vi "imp_test_v12_p.vi"() -> ()   [LabVIEW 2014]
uses:
  <vilib>/LabVIEW Targets/FPGA/cRIO/shared/nicrio_ModuleControls/nicrio_cRIO-9237_DataRatesRing.ctl
  <vilib>/LabVIEW Targets/FPGA/cRIO/shared/nicrio_ModuleControls/nicrio_cRIO-9237_ExcitationVoltageRing.ctl
  <vilib>/rvi/FXPMathLib/FxpSinAndCos/subVIs/nifxpmath_SinAndCos_SimConfig.ctl
  <vilib>/rvi/FXPMathLib/FxpSqrt/subVIs/nifxpmath_Sqrt_SimConfig.ctl
  <vilib>/fxp/LVFixedPointOverflowPolicyTypeDef.ctl
  <vilib>/rvi/FXPMathLib/FxpAtan2/subVIs/nifxpmath_Atan2_SimConfig.ctl
  <vilib>/rvi/Emulation/niFpgaGetClockAttributes.vi
  <vilib>/rvi/Emulation/niFpgaSctlEmulationGetInTimedLoop.vi
  <vilib>/rvi/Emulation/niFpgaEmulationReportErrorSimple.vi
  <vilib>/rvi/Emulation/niFpgaProcessEmulError.vi
  <vilib>/rvi/interface/RandomDataEmulation/nirviRandomDataMultiElementFPGAFIFO.vi
  <instcachedir>/0/nirviRandomDataMultiElementFPGAFIFO_AD0CFC12EF974623A9C2E4184BC062B2.lvgen/nirviRandomDataMultiElementFPGAFIFO_AD0CFC12EF974623A9C2E4184BC062B2_028.vi
  <vilib>/rvi/interface/RandomDataEmulation/niFpgaRandomDataHandleErrors.vi
  <vilib>/rvi/Emulation/niFpgaCriticalErrorInLSC.vi
  <vilib>/rvi/FXPMathLib/FxpSinAndCos/simVIs/DllFxpSinAndCosTemp_sub.vi
  <vilib>/rvi/eio/common/nirviEmuTemplateMethod_errors.vi
  <vilib>/rvi/FXPMathLib/FxpSqrt/simVIs/DllSqrtTemp_sub.vi
  <vilib>/rvi/FXPMathLib/FxpAtan2/simVIs/DllFxpAtan2Temp_sub.vi
  <vilib>/rvi/eio/common/nirviEmuTemplatePropertySet_errors.vi
  <vilib>/rvi/DataTransferAndStorage/Container/XNode/niFpgaContainer.xnode
  <vilib>/rvi/interface/RandomDataEmulation/nirviRandomDataFpgaMultiElementTemplate.vi
  <vilib>/rvi/Analysis/measure/butterworth/XNode/niFpgaButterworthFilter.xnode
  <vilib>/rvi/FXPMathLib/FxpSinAndCos/XNode/nifxpmath_SinAndCos.xnode
  <vilib>/eio/EIONode/EIONode.xnode
  <vilib>/rvi/FXPMathLib/FxpSqrt/XNode/nifxpmath_Sqrt.xnode
  <vilib>/rvi/FXPMathLib/FxpAtan2/XNode/nifxpmath_Atan2.xnode
  <vilib>/eio/EIOPropertyNode/EIOPropertyNode.xnode
  <vilib>/rvi/eio/common/nirviEmuTemplatePropertyGet_errors.vi
  <vilib>/rvi/eio/common/nirviEmuTemplatePropertyGet_noerrors.vi
  <vilib>/rvi/eio/common/nirviEmuTemplatePropertySet_noerrors.vi
panel:
  out "(b^2-ac)p3":fxp<+/-,64,35>
  out "(b^2-ac)p2":fxp<+/-,64,34>
  in  "kv_p (Nm/rad)":fxp<+/-,32,7>
  out "tau_p (Nm)":fxp<+/-,53,16>
  out "theta3p (rad)":fxp<+/-,19,5>
  out "theta2p (rad)":fxp<+/-,16,2>
  out "r4p":fxp<+/-,32,9>
  in  "force_lim":fxp<+,22,9>
  in  "Mavg f loop(uSec)":u32
  in  "F_Threshold_p":fxp<+,12,4>
  out "omega_p (Mavg)":fxp<+/-,36,13>
  out "Dp_d (Mavg)":fxp<+/-,36,13>
  out "omega_p2 (Mavg)":fxp<+/-,36,14>
  out "Dp2_d (Mavg)":fxp<+/-,36,14>
  in  "mt0_p2":u32
  out "Dp_d (Mavg w. f.)":fxp<+/-,36,14>
  in  "Dp_d (Mavg) coeff.":i32[](array[numeric])=[946630756, 63555534]
  out "omega_p (Mavg w. f)":fxp<+/-,36,14>
  in  "omega_P(Mavg) coeff.":i32[](array[numeric])=[946630756, 63555534]
  out "PID (kHz)":fxp<+/-,20,10>
  in  "Set 6":bool
  in  "Set 5":bool
  in  "Set 4":bool
  in  "Set 3":bool
  in  "Set 2":bool
  in  "Set 1":bool
  out "Dp1_d (T)":fxp<+/-,36,13>
  out "omega_p1 (T)":fxp<+/-,36,13>
  out "Dp2_d (T)":fxp<+/-,36,13>
  out "omega_p2 (T)":fxp<+/-,36,13>
  out "mt_omega_p2":u32
  out "Encoder Position_p2":i32
  out "D_p2":fxp<+/-,32,7>
  out "rad_p2":fxp<+/-,33,20>
  out "D_p1":fxp<+/-,32,7>
  out "rad_p1":fxp<+/-,33,20>
  out "Encoder Position_p1":i32
  out "Dp1_d (Mavg)":fxp<+/-,36,14>
  out "omega_p1 (Mavg)":fxp<+/-,36,14>
  in  "Dp_d_M_avg_Tc (uSec)":i32
  out "Dp_d (T)":fxp<+/-,36,13>
  out "omega_p (T)":fxp<+/-,36,13>
  in  "Vp. Est.":i16(ring) items=["T", "Mavg", "Mavg w. f."]
  in  "Mag. factor_p":fxp<+/-,20,3>
  in  "Mag. encoder_p":bool
  in  "Belt_out_p":fxp<+/-,7,7>
  in  "Belt_in_p":fxp<+/-,6,6>
  out "Fp_dc":fxp<+/-,32,10>
  in  "Zero_p":bool
  in  "mt0_p1":u32
  in  "Encoder reset":bool
  out "fpt_d":fxp<+/-,36,18>
  out "Dp_error_dd":fxp<+/-,36,16>
  out "Dp_error_d":fxp<+/-,33,8>
  in  "Dp_dd coeff.":i32[](array[numeric])=[946630756, 63555534]
  out "Dp_dd":fxp<+/-,36,25>
  out "dFp_PID":fxp<+/-,36,18>
  in  "dFp_PID coeff.":i32[](array[numeric])=[946630756, 63555534]
  out "fpt_i":fxp<+/-,34,18>
  in  "Bv_p":fxp<+/-,22,8>
  in  "Kv_p":fxp<+/-,26,7>
  out "Dp_error":fxp<+/-,22,7>
  out "Dpr_sin":fxp<+/-,22,7>
  in  "Sin offset_p":fxp<+/-,22,7>
  in  "Sin magnitude_p":fxp<+/-,21,6>
  out "Dpr_sin_dd":fxp<+/-,35,20>
  out "Dpr_sin_d":fxp<+/-,33,15>
  out "Sin omega_p":fxp<+/-,34,9>
  in  "Sin wave freq._p (Hz)":fxp<+/-,32,6>
  in  "Dpr_step":fxp<+/-,22,7>
  out "Dpr_for":fxp<+/-,22,7>
  in  "Command_p":i16(ring) items=["Step", "Sine"]
  in  "Ki_p":fxp<+/-,30,9>
  out "Fp_PID":fxp<+/-,36,16>
  in  "fp_tolorance":fxp<+,22,6>
  out "fp_tilde":fxp<+/-,33,10>
  in  "Kd_p":fxp<+/-,30,9>
  in  "Kp_p":fxp<+/-,32,13>
  out "Fr_p":fxp<+/-,32,10>
  in  "S/F coeff_p":fxp<+/-,25,-10>
  out "va_p":fxp<+/-,36,7>
  out "vb_p":fxp<+/-,37,8>
  out "vq_p_F":fxp<+/-,20,5> format="%.57g"
  out "vd_p_F":fxp<+/-,20,5>
  in  "dFp_add":bool
  in  "Stop motor_p":bool
  out "Force_p":fxp<+/-,32,10>
  in  "Strain selection_p":i16(ring) items=["Raw", "Avg.8", "Avg.8 w. filter"]
  out "Strain_p (Avg8 w. f)":fxp<+/-,36,8>
  in  "Strain_p Avg.8 coeff.":i32[](array[numeric])=[946630756, 63555534]
  out "Strain_p (Avg8)":fxp<+/-,36,4>
  out "Raw Strain_p":fxp<+/-,36,4>
  out "Mod6/AI3":fxp<+/-,36,4>
  in  "Strain gage reset_p":bool
  out "Dp_d (mm/s)":fxp<+/-,36,13>
  out "omega_p (rad/s)":fxp<+/-,36,13>
  out "mt_omega_p1":u32
  out "rad_p(NrTheta)":fxp<+/-,33,20>
  out "D_p(mm)":fxp<+/-,32,7>
  out "Encoder Position_p":i32
  in  "Encoder reset_p":bool
  out "Time now(s)":fxp<+,52,14>
  in  "Drive mode":i16(ring) items=["Backward", "Forward", "Imp", "Imp(tau2theta)"]
  in  "Ini coe.":bool
  out "Loop rate (kHz)":fxp<+/-,36,7>
  in  "Stop (Strain)":bool
  in  "Excitation Voltage":T1 items=["2.5 Volts", "3.3 Volts", "5.0 Volts", "10.0 Volts", "External Excitation"]
  in  "Data Rate":T2=1 items=["50.000 kS/s (NI 9237)"=1, "25.000 kS/s (NI 9237)"=2, "16.667 kS/s (NI 9237)"=3, "12.500 kS/s (NI 9237)"=4, "10.000 kS/s (NI 9237)"=5, "8.333 kS/s (NI 9237)"=6, "7.143 kS/s (NI 9237)"=7, "6.250 kS/s (NI 9237)"=8, "5.556 kS/s (NI 9237)"=9, "5.000 kS/s (NI 9237)"=10, "4.545 kS/s (NI 9237)"=11, "4.167 kS/s (NI 9237)"=12, "3.846 kS/s (NI 9237)"=13, "3.571 kS/s (NI 9237)"=14, "3.333 kS/s (NI 9237)"=15, "3.125 kS/s (NI 9237)"=16, "2.941 kS/s (NI 9237)"=17, "2.778 kS/s (NI 9237)"=18, "2.632 kS/s (NI 9237)"=19, "2.500 kS/s (NI 9237)"=20, "2.381 kS/s (NI 9237)"=21, "2.273 kS/s (NI 9237)"=22, "2.174 kS/s (NI 9237)"=23, "2.083 kS/s (NI 9237)"=24, "2.000 kS/s (NI 9237)"=25, "1.923 kS/s (NI 9237)"=26, "1.852 kS/s (NI 9237)"=27, "1.786 kS/s (NI 9237)"=28, "1.724 kS/s (NI 9237)"=29, "1.667 kS/s (NI 9237)"=30, "1.613 kS/s (NI 9237)"=31]
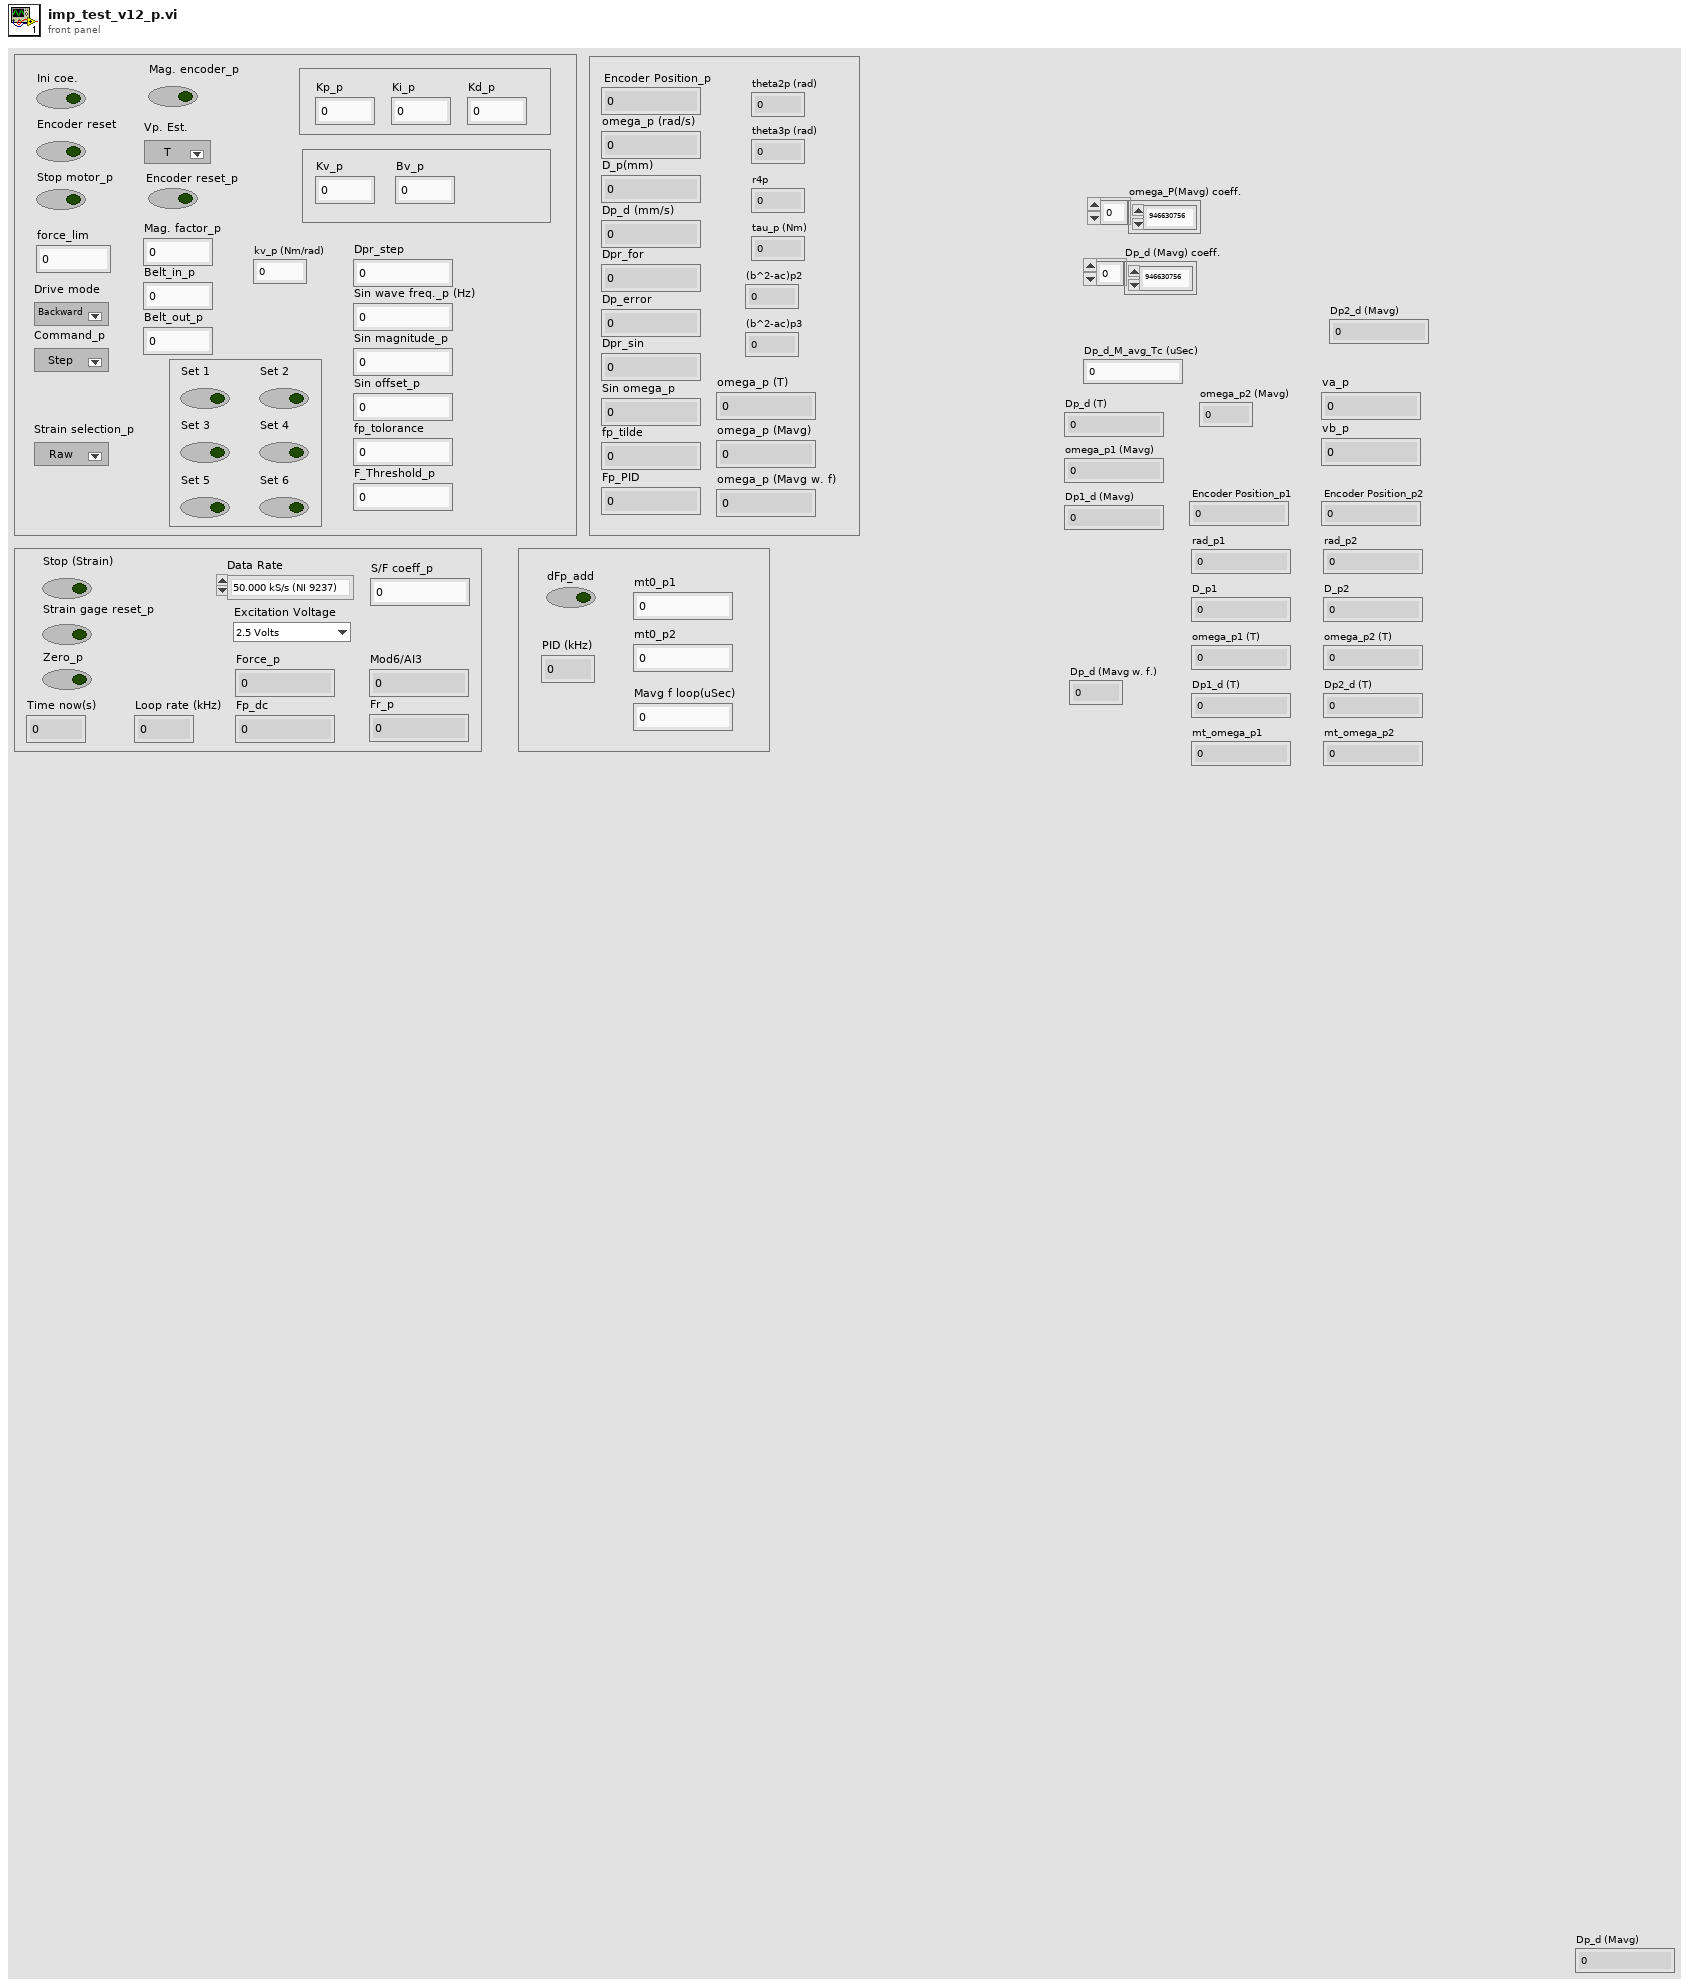
[diagram p1: front panel]
types:
  T1 = typedef "nicrio_cRIO-9237_ExcitationVoltageRing.ctl" = u8
  T2 = typedef "nicrio_cRIO-9237_DataRatesRing.ctl" = u8
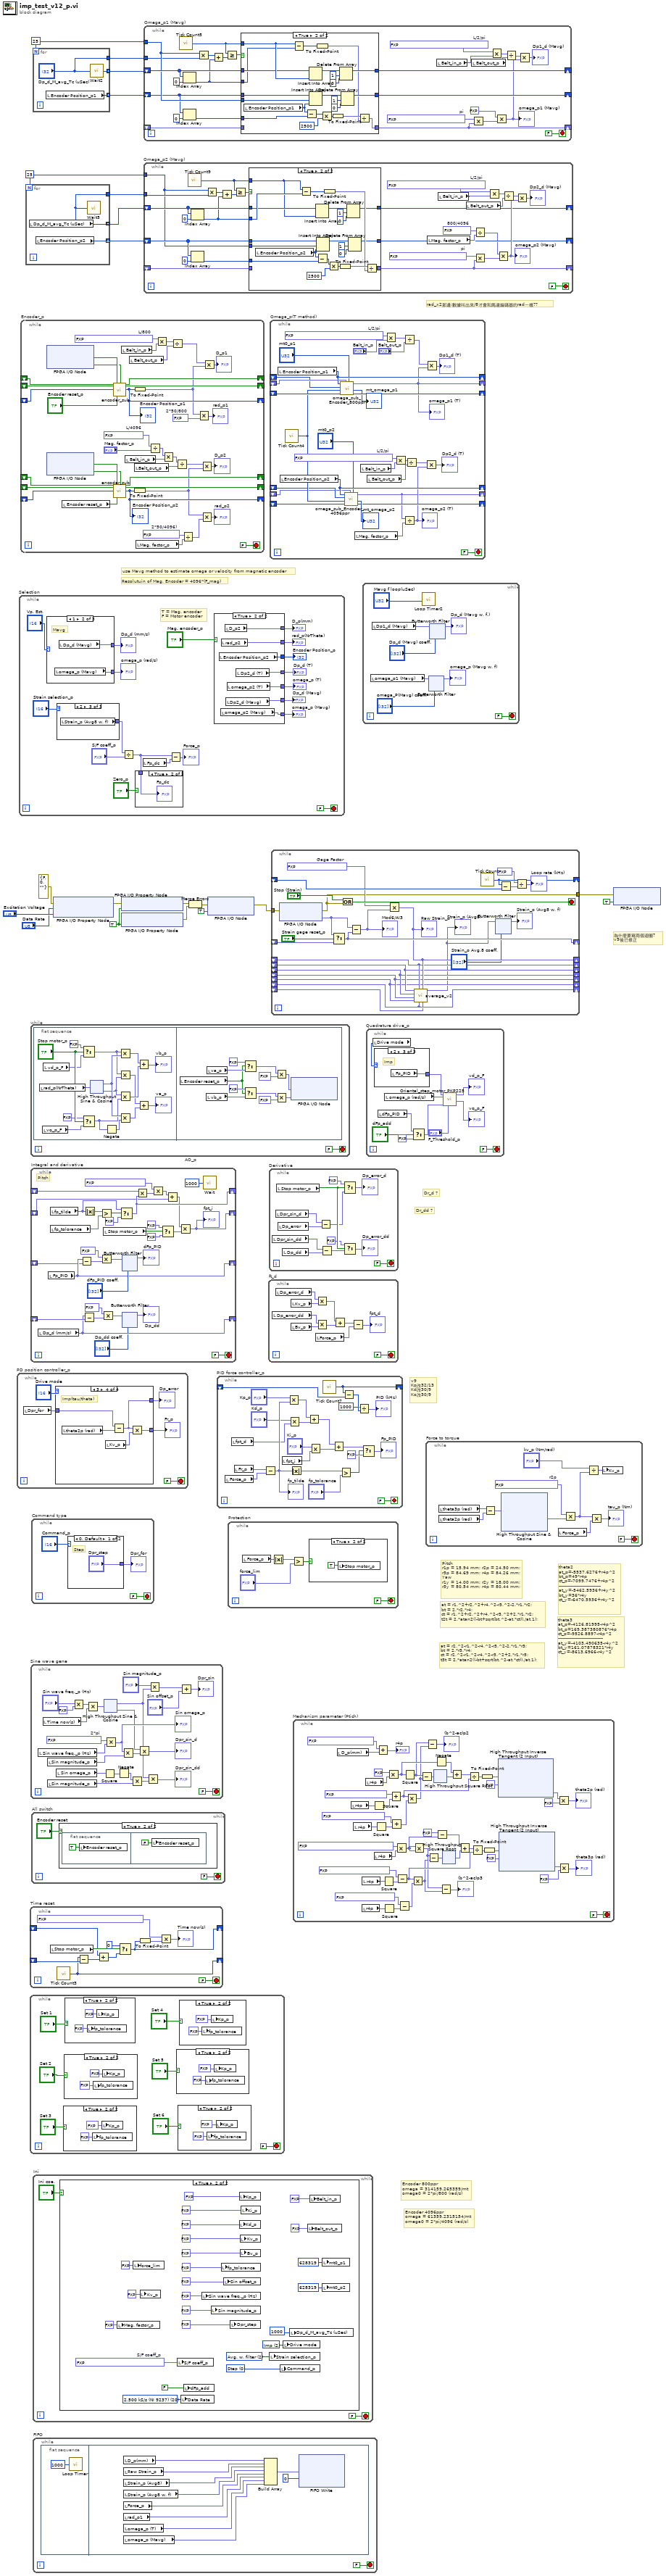
[diagram p0: block diagram]
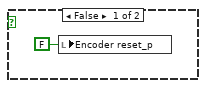
[diagram p11: hidden frame]
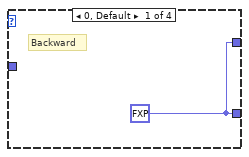
[diagram p12: hidden frame]
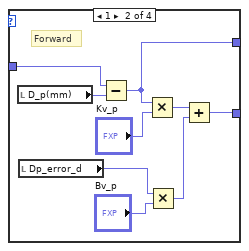
[diagram p13: hidden frame]
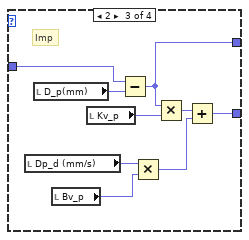
[diagram p14: hidden frame]
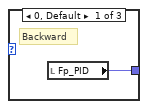
[diagram p15: hidden frame]
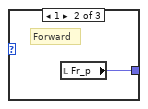
[diagram p16: hidden frame]
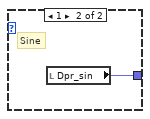
[diagram p17: hidden frame]
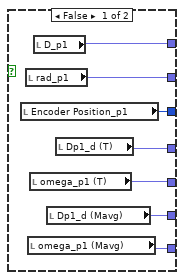
[diagram p18: hidden frame]
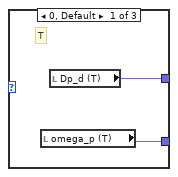
[diagram p19: hidden frame]
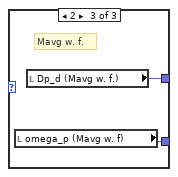
[diagram p20: hidden frame]
diagram:
  w2 = 25
  w8 = 25
  w13 = TRUE ("Half-Bridge Enable")
  # "theta3\nat_p=-4126.81995-r4p^2\nbt_p=169.387380876*r4p\nct_p=-9526.8897-r4p^2\n-------------------------------\nat_y=-4103.490635-r4y^2\nbt_y=161.07878321*r4y\nct_y=-8613.6966-r4y^2"
  # "at = r2.^2-r1.^2-r4.^2-r3.^2-2.*r1.*r3;\nbt = 2.*r3.*r4;\nct = r2.^2-r1.^2-r4.^2-r3.^2+2.*r1.*r3;\nt3t = 2.*atan2((-bt+sqrt(bt.^2-at.*ct))./at,1);"
  # "theta2\nat_p=-5537.6276+r4p^2\nbt_p=49*r4p\nct_p=-7099.7476+r4p^2\n-----------------------------\nat_y=-5462.5936+r4y^2\nbt_y=36*r4y\nct_y=-6470.5936+r4y^2"
  # "Pitch\nr1p = 15.94 mm; r2p = 24.50 mm;\nr3p = 84.69 mm; r4p = 84.26 mm;\nYaw\nr1y = 14.00 mm; r2y = 18.00 mm;\nr3y = 80.54 mm; r4p = 80.44 mm;"
  # "at = r1.^2+r2.^2+r4.^2-r3.^2-2.*r1.*r2;\nbt = 2.*r2.*r4;\nct = r1.^2+r2.^2+r4.^2-r3.^2+2.*r1.*r2;\nt2t = 2.*atan2((-bt+sqrt(bt.^2-at.*ct))./at,1);"
  # "rad_x2那邊:數據叫出來/8才會和馬達編碼器的rad一樣??"
  # "Encoder 4096ppr\nomega = 61359.2315154/mt\nomega0 = 2*pi/4096 (rad/s)"
  # "Encoder 800ppr\nomega = 314159.265359/mt\nomega0 = 2*pi/800 (rad/s)"
  # "v9\nKp改32/13\nKd改30/9\nKo改30/9"
  # "Resolutuin of Mag. Encoder = 4096*(F_mag)"
  # "use Mavg method to estimate omega or velocity from magnetic encoder"
  # "為什麼要寫兩個迴圈?\nv9後已修正"
  # "Dr_dd ?"
  # "Dr_d ?"
  n1 = while "PD position controller_p" {
    stop <- FALSE stop-if-true
    n2 = local read "Dpr_for"() -> (w21:fxp<+/-,22,7>)
    n3 = case shown="3" "Drive mode" {
      tunnel: [w26 w30 w37 w45] -> w25
      tunnel: [w26 w28 w42 w47] -> w22
      tunnel: w21 -> [_ w27 w36 w46]
      frame 0, Default {
        w26 = fxp<+/-,62,19> 0.0
        # "Backward"
      }
      frame 1 {
        # "Forward"
        n4 = local read "D_p(mm)"() -> (w35:fxp<+/-,32,7>)
        n5 = local read "Dp_error_d"() -> (w29:fxp<+/-,33,8>)
        n6 = Subtract(x=w27, y=w35) -> (x-y=w28:fxp<+/-,33,8>)
        n7 = Multiply(x=w28, y="Kv_p") -> (x*y=w32:fxp<+/-,58,14>)
        n8 = Multiply(x=w29, y="Bv_p") -> (x*y=w31:fxp<+/-,55,16>)
        n9 = Add(x=w32, y=w31) -> (x+y=w30:fxp<+/-,60,16>)
      }
      frame 2 {
        # "Imp"
        n10 = local read "Dp_d (mm/s)"() -> (w40:fxp<+/-,36,13>)
        n11 = local read "D_p(mm)"() -> (w43:fxp<+/-,32,7>)
        n12 = local read "Bv_p"() -> (w39:fxp<+/-,22,8>)
        n13 = local read "Kv_p"() -> (w44:fxp<+/-,26,7>)
        n14 = Subtract(x=w36, y=w43) -> (x-y=w42:fxp<+/-,33,8>)
        n15 = Multiply(x=w40, y=w39) -> (x*y=w38:fxp<+/-,58,21>)
        n16 = Multiply(x=w42, y=w44) -> (x*y=w41:fxp<+/-,58,14>)
        n17 = Add(x=w41, y=w38) -> (x+y=w37:fxp<+/-,64,21>)
      }
      frame 3 {
        # "Imp(tau/theta)"
        n18 = local read "theta2p (rad)"() -> (w48:fxp<+/-,16,2>)
        n19 = local read "Kv_p"() -> (w49:fxp<+/-,26,7>)
        n20 = Subtract(x=w46, y=w48) -> (x-y=w47:fxp<+/-,23,8>)
        n21 = Multiply(x=w47, y=w49) -> (x*y=w45:fxp<+/-,48,14>)
      }
    }
    "Fr_p" <- w25
    "Dp_error" <- w22
  }
  n22 = while "Selection" {
    stop <- FALSE stop-if-true
    # "T = Mag. encoder\nF = Motor encoder"
    n23 = case shown="1" "Vp. Est." {
      tunnel: [w84 w85 w88] -> w60
      tunnel: [w83 w86 w87] -> w61
      frame 0, Default {
        # "T"
        n24 = local read "omega_p (T)"() -> (w84:fxp<+/-,36,13>)
        n25 = local read "Dp_d (T)"() -> (w83:fxp<+/-,36,13>)
      }
      frame 1 {
        # "Mavg"
        n26 = local read "omega_p (Mavg)"() -> (w85:fxp<+/-,36,13>)
        n27 = local read "Dp_d (Mavg)"() -> (w86:fxp<+/-,36,13>)
      }
      frame 2 {
        # "Mavg w. f."
        n28 = local read "omega_p (Mavg w. f)"() -> (w88:fxp<+/-,36,14>)
        n29 = local read "Dp_d (Mavg w. f.)"() -> (w87:fxp<+/-,36,14>)
      }
    }
    "Dp_d (mm/s)" <- w61
    "omega_p (rad/s)" <- w60
    n30 = case shown="2" "Strain selection_p" {
      tunnel: [w90 w91 w92] -> w67
      frame 0, Default {
        n31 = local read "Raw Strain_p"() -> (w90:fxp<+/-,36,4>)
      }
      frame 1 {
        n32 = local read "Strain_p (Avg8)"() -> (w91:fxp<+/-,36,4>)
      }
      frame 2 {
        n33 = local read "Strain_p (Avg8 w. f)"() -> (w92:fxp<+/-,36,8>)
      }
    }
    n34 = Divide(x=w67, y="S/F coeff_p") -> (x/y=w64:fxp<+/-,32,10>)
    n35 = case shown="True" "Zero_p" {
      tunnel: w64 -> [_ w89]
      frame False {
      }
      frame True {
        "Fp_dc" <- w89
      }
    }
    n36 = local read "Fp_dc"() -> (w62:fxp<+/-,32,10>)
    n37 = Subtract(x=w64, y=w62) -> (x-y=→"Force_p":fxp<+/-,33,11>)
    n38 = case shown="True" "Mag. encoder_p" {
      tunnel: [w75 w82] -> w56
      tunnel: [w74 w81] -> w57
      tunnel: [w73 w80] -> w58
      tunnel: [w71 w79] -> w54
      tunnel: [w72 w78] -> w53
      tunnel: [w70 w76] -> w52
      tunnel: [w69 w77] -> w51
      frame False {
        n39 = local read "Encoder Position_p1"() -> (w73:i32)
        n40 = local read "rad_p1"() -> (w74:fxp<+/-,33,20>)
        n41 = local read "omega_p1 (Mavg)"() -> (w69:fxp<+/-,36,14>)
        n42 = local read "omega_p1 (T)"() -> (w71:fxp<+/-,36,13>)
        n43 = local read "D_p1"() -> (w75:fxp<+/-,32,7>)
        n44 = local read "Dp1_d (Mavg)"() -> (w70:fxp<+/-,36,14>)
        n45 = local read "Dp1_d (T)"() -> (w72:fxp<+/-,36,13>)
      }
      frame True {
        n46 = local read "Encoder Position_p2"() -> (w80:i32)
        n47 = local read "omega_p2 (Mavg)"() -> (w77:fxp<+/-,36,14>)
        n48 = local read "rad_p2"() -> (w81:fxp<+/-,33,20>)
        n49 = local read "D_p2"() -> (w82:fxp<+/-,32,7>)
        n50 = local read "Dp2_d (Mavg)"() -> (w76:fxp<+/-,36,14>)
        n51 = local read "omega_p2 (T)"() -> (w79:fxp<+/-,36,13>)
        n52 = local read "Dp2_d (T)"() -> (w78:fxp<+/-,36,13>)
      }
    }
    "D_p(mm)" <- w56
    "rad_p(NrTheta)" <- w57
    "Encoder Position_p" <- w58
    "Dp_d (T)" <- w53
    "omega_p (T)" <- w54
    "Dp_d (Mavg)" <- w52
    "omega_p (Mavg)" <- w51
  }
  n53 = while "Encoder_p" {
    shift-right: [w130] -> _
    shift-left: _ -> [w129]
    shift-right: [w131] -> _
    shift-left: _ -> [w128]
    shift-right: [w125] -> _
    shift-left: _ -> [w127]
    shift-right: [w116] -> _
    shift-left: _ -> [w115]
    shift-right: [w117] -> _
    shift-left: _ -> [w118]
    shift-right: [w112] -> _
    shift-left: _ -> [w113]
    stop <- FALSE stop-if-true
    w108 = fxp<+/-,20,-5> 0.00048828125  # L/4096
    w106 = fxp<+/-,16,1> 0.0244140625  # 2*50/4096)
    w124 = fxp<+/-,20,-5> 0.002499997615814209  # L/800
    w98 = fxp<+/-,16,1> 0.125  # 2*50/800
    n54 = xnode "FPGA I/O Node"() -> ("Mod7/DIO0"=w133:bool, "Mod7/DIO1"=w132:bool)  [unwired: 2 in, 2 out]
    n55 = xnode "FPGA I/O Node"() -> ("Mod7/DIO4"=w120:bool, "Mod7/DIO5"=w119:bool)  [unwired: 2 in, 2 out]
    n56 = local read "Encoder reset_p"() -> (w114:bool)
    n57 = call "encoder_sub.vi"("A_pre"=w129, "B_pre"=w128, "Encoder Position_pre"=w127, "A input"=w133, "Encoder Position Reset"="Encoder reset_p", "B input"=w132) -> ("A"=w130:bool, "B"=w131:bool, "Encoder Position (Counts)"=w125:i32)  [unwired: 19 in]
    "Encoder Position_p1" <- w125
    n58 = call "encoder_sub.vi"("A_pre"=w115, "B_pre"=w118, "Encoder Position_pre"=w113, "A input"=w120, "Encoder Position Reset"=w114, "B input"=w119) -> ("A"=w116:bool, "B"=w117:bool, "Encoder Position (Counts)"=w112:i32)  [unwired: 19 in]
    "Encoder Position_p2" <- w112
    n59 = local read "Belt_in_p"() -> (w123:fxp<+/-,6,6>)
    n60 = local read "Belt_in_p"() -> (w109:fxp<+/-,6,6>)
    n61 = local read "Belt_out_p"() -> (w121:fxp<+/-,7,7>)
    n62 = To Fixed-Point(number=w112) -> (fixed-point=w94:fxp<+/-,32,32>)  [unwired: 1 in]
    n63 = To Fixed-Point(number=w125) -> (fixed-point=w99:fxp<+/-,32,32>)  [unwired: 1 in]
    n64 = local read "Belt_out_p"() -> (w111:fxp<+/-,7,7>)
    n65 = local read "Mag. factor_p"() -> (w105:fxp<+/-,20,3>)
    n66 = Divide(x=w108, y="Mag. factor_p") -> (x/y=w107:fxp<+/-,41,13>)
    n67 = Multiply(x=w124, y=w123) -> (x*y=w122:fxp<+/-,26,1>)
    n68 = Multiply(x=w107, y=w109) -> (x*y=w110:fxp<+/-,46,18>)
    n69 = Divide(x=w122, y=w121) -> (x/y=w101:fxp<+/-,33,1>)
    n70 = Divide(x=w110, y=w111) -> (x/y=w96:fxp<+/-,53,18>)
    n71 = Divide(x=w106, y=w105) -> (x/y=w93:fxp<+/-,37,5>)
    n72 = Multiply(x=w99, y=w98) -> (x*y=→"rad_p1":fxp<+/-,33,20>)
    n73 = Multiply(x=w96, y=w94) -> (x*y=→"D_p2":fxp<+/-,37,7>)
    n74 = Multiply(x=w94, y=w93) -> (x*y=→"rad_p2":fxp<+/-,46,16>)
    n75 = Multiply(x=w101, y=w99) -> (x*y=→"D_p1":fxp<+/-,32,7>)
  }
  n76 = for {
    N: w2 -> [_]
    tunnel: [w135] -> w4 mode=indexing
    tunnel: [w134] -> w3 mode=indexing
    tunnel: [w134] -> w1
    n77 = local read "Dp_d_M_avg_Tc (uSec)"() -> (w134:i32)
    n78 = local read "Encoder Position_p2"() -> (w135:i32)
    n79 = call "Wait5"("Count(uSec)"=w134) -> ()  [unwired: 1 out]
  }
  n80 = while "Time reset" {
    shift-right: [w145] -> _
    shift-left: _ -> [w146]
    shift-right: [w140] -> _
    shift-left: _ -> [w141]
    stop <- FALSE stop-if-true
    n81 = local read "Stop motor_p"() -> (w147:bool)
    n82 = call "Tick Count3"() -> ("Tick Count(uSec)"=w145:u32)
    n83 = Subtract(x=w145, y=w146) -> (x-y=w144:u32)
    n84 = Add(x=w141, y=w144) -> (x+y=w143:u32)
    n85 = Select(t=u32 0, s=w147, f=w143) -> (s? t:f=w140:u32)
    n86 = To Fixed-Point(number=w140) -> (fixed-point=w139:fxp<+,32,32>)  [unwired: 1 in]
    n87 = Multiply(x=fxp<+,20,-18> 1.0000003385357559e-06, y=w139) -> (x*y=→"Time now(s)":fxp<+,52,14>)
  }
  n88 = while {
    stop <- FALSE stop-if-true
    n89 = case shown="True" "Set 3" {
      frame False {
      }
      frame True {
        n90 = local write "fp_tolorance"(fxp<+,22,6> 3.0 ("fp_tolorance")) -> ()
        n91 = local write "Kp_p"(fxp<+/-,36,9> 100.0 ("Kp_p")) -> ()
      }
    }
    n92 = case shown="True" "Set 2" {
      frame False {
      }
      frame True {
        n93 = local write "fp_tolorance"(fxp<+,22,6> 1.5 ("fp_tolorance")) -> ()
        n94 = local write "Kp_p"(fxp<+/-,36,9> 50.0 ("Kp_p")) -> ()
      }
    }
    n95 = case shown="True" "Set 1" {
      frame False {
      }
      frame True {
        n96 = local write "fp_tolorance"(fxp<+,22,6> 3.0 ("fp_tolorance")) -> ()
        n97 = local write "Kp_p"(fxp<+/-,36,9> 50.0 ("Kp_p")) -> ()
      }
    }
    n98 = case shown="True" "Set 5" {
      frame False {
      }
      frame True {
        n99 = local write "fp_tolorance"(fxp<+,22,6> 3.0 ("fp_tolorance")) -> ()
        n100 = local write "Kp_p"(fxp<+/-,36,9> 150.0 ("Kp_p")) -> ()
      }
    }
    n101 = case shown="True" "Set 6" {
      frame False {
      }
      frame True {
        n102 = local write "fp_tolorance"(fxp<+,22,6> 1.5 ("fp_tolorance")) -> ()
        n103 = local write "Kp_p"(fxp<+/-,36,9> 150.0 ("Kp_p")) -> ()
      }
    }
    n104 = case shown="True" "Set 4" {
      frame False {
      }
      frame True {
        n105 = local write "fp_tolorance"(fxp<+,22,6> 1.5 ("fp_tolorance")) -> ()
        n106 = local write "Kp_p"(fxp<+/-,36,9> 100.0 ("Kp_p")) -> ()
      }
    }
  }
  n107 = while "AO_p" {
    stop <- FALSE stop-if-true
    n108 = flat-sequence {
      frame #0 {
        n109 = local read "rad_p(NrTheta)"() -> (w179:fxp<+/-,33,20>)
        n110 = local read "vq_p_F"() -> (w180:fxp<+/-,20,5>)
        n111 = local read "vd_p_F"() -> (w182:fxp<+/-,20,5>)
        n112 = Select(t=fxp<+/-,20,5> 0.0, s="Stop motor_p", f=w182) -> (s? t:f=w171:fxp<+/-,20,5>)
        n113 = Select(t=fxp<+,1,1> 0.0, s="Stop motor_p", f=w180) -> (s? t:f=w170:fxp<+/-,20,5>)
        n114 = xnode "High Throughput Sine & Cosine"("x (pi)"=w179) -> ("sin(x)"=w173:fxp<+/-,16,2>, "cos(x)"=w172:fxp<+/-,16,2>)
        n115 = Negate(x=w170) -> (-x=w178:fxp<+/-,21,6>)
        n116 = Multiply(x=w171, y=w173) -> (x*y=w177:fxp<+/-,36,7>)
        n117 = Multiply(x=w171, y=w172) -> (x*y=w175:fxp<+/-,36,7>)
        n118 = Multiply(x=w172, y=w170) -> (x*y=w176:fxp<+/-,36,7>)
        n119 = Multiply(x=w173, y=w178) -> (x*y=w174:fxp<+/-,35,6>)
        n120 = Add(x=w177, y=w176) -> (x+y=→"vb_p":fxp<+/-,37,8>)
        n121 = Add(x=w175, y=w174) -> (x+y=→"va_p":fxp<+/-,36,7>)
      }
      frame #1 {
        n122 = local read "Encoder reset_p"() -> (w215:bool)
        n123 = local read "vb_p"() -> (w216:fxp<+/-,37,8>)
        n124 = local read "va_p"() -> (w217:fxp<+/-,36,7>)
        n125 = Select(t=fxp<+,2,2> 3.0, s=w215, f=w217) -> (s? t:f=w223:fxp<+/-,36,7>)
        n126 = Select(t=fxp<+,1,1> 0.0, s=w215, f=w216) -> (s? t:f=w222:fxp<+/-,37,8>)
        n127 = Multiply(x=w223, y=fxp<+/-,1,0> -0.5) -> (x*y=w218:fxp<+/-,36,6>)
        n128 = Multiply(x=w222, y=fxp<+/-,1,0> -0.5) -> (x*y=w219:fxp<+/-,36,6>)
        n129 = xnode "FPGA I/O Node"("Mod8/AO0"=w218, "Mod8/AO1"=w219) -> ()  [unwired: 2 in, 2 out]
      }
    }
  }
  n130 = while "Sine wave gene" {
    stop <- FALSE stop-if-true
    w231 = fxp<+,20,3> 6.2831878662109375  # 2*pi
    n131 = local read "Sin wave freq._p (Hz)"() -> (w227:fxp<+/-,32,6>)
    n132 = local read "Time now(s)"() -> (w245:fxp<+,52,14>)
    n133 = local read "Sin magnitude_p"() -> (w228:fxp<+/-,21,6>)
    n134 = local read "Sin magnitude_p"() -> (w230:fxp<+/-,21,6>)
    n135 = local read "Sin omega_p"() -> (w229:fxp<+/-,34,9>)
    n136 = Multiply(x="Sin wave freq._p (Hz)", y=fxp<+/-,10,3> 2.0) -> (x*y=w249:fxp<+/-,42,9>)
    n137 = Multiply(x=w249, y=w245) -> (x*y=w246:fxp<+/-,41,19>)
    n138 = Square(x=w229) -> (x^2=w241:fxp<+,34,18>)
    n139 = xnode "High Throughput Sine & Cosine"("x (pi)"=w246) -> ("sin(x)"=w232:fxp<+/-,16,2>, "cos(x)"=w237:fxp<+/-,16,2>)
    n140 = Multiply(x=w231, y=w227) -> (x*y=w244:fxp<+/-,34,9>)
    "Sin omega_p" <- w244
    n141 = Negate(x=w241) -> (-x=w240:fxp<+/-,35,19>)
    n142 = Multiply(x=w244, y=w228) -> (x*y=w243:fxp<+/-,33,15>)
    n143 = Multiply(x=w240, y=w230) -> (x*y=w239:fxp<+/-,35,19>)
    n144 = Multiply(x=w237, y=w243) -> (x*y=→"Dpr_sin_d":fxp<+/-,33,15>)
    n145 = Multiply(x=w232, y=w239) -> (x*y=→"Dpr_sin_dd":fxp<+/-,35,20>)
    n146 = Multiply(x="Sin magnitude_p", y=w232) -> (x*y=w235:fxp<+/-,37,8>)
    n147 = Add(x=w235, y="Sin offset_p") -> (x+y=→"Dpr_sin":fxp<+/-,37,8>)
  }
  n148 = while "Integral and derivative" {
    shift-right: [w303] -> _
    shift-left: _ -> [w306]
    shift-right: [w296] -> _
    shift-left: _ -> [w295]
    shift-right: [w290] -> _
    shift-left: _ -> [w289]
    shift-right: [w285] -> _
    shift-left: _ -> [w286]
    stop <- FALSE stop-if-true
    # "Pitch"
    n149 = local read "Dp_d (mm/s)"() -> (w285:fxp<+/-,36,13>)
    n150 = local read "Fp_PID"() -> (w290:fxp<+/-,36,16>)
    n151 = local read "fp_tilde"() -> (w307:fxp<+/-,33,10>)
    n152 = local read "fp_tolorance"() -> (w310:fxp<+,22,6>)
    n153 = Subtract(x=w290, y=w289) -> (x-y=w294:fxp<+/-,37,17>)
    n154 = Subtract(x=w285, y=w286) -> (x-y=w287:fxp<+/-,37,14>)
    n155 = Absolute Value(x=w307) -> (abs(x)=w311:fxp<+,33,10>)
    n156 = Greater?(x=w311, y=w310) -> (0:w309:bool)
    n157 = Multiply(x=fxp<+,7,10> 1000.0, y=w294) -> (x*y=w292:fxp<+/-,32,18>)
    n158 = Multiply(x=fxp<+,7,10> 1000.0, y=w287) -> (x*y=w283:fxp<+/-,36,21>)
    n159 = local read "Stop motor_p"() -> (w298:bool)
    n160 = Select(t=w307, s=w309, f=fxp<+,1,1> 0.0) -> (s? t:f=w303:fxp<+/-,33,10>)
    n161 = xnode "Butterworth Filter"("input data"=w292, "scaled coefficients"="dFp_PID coeff.") -> ("output data"=→"dFp_PID":fxp<+/-,36,22>)  [unwired: 1 in]
    n162 = xnode "Butterworth Filter"("input data"=w283, "scaled coefficients"="Dp_dd coeff.") -> ("output data"=→"Dp_dd":fxp<+/-,36,25>)  [unwired: 1 in]
    n163 = Multiply(x=w306, y=w303) -> (x*y=w305:fxp<+/-,34,12>)
    n164 = Multiply(x=fxp<+/-,30,12> 0.000499725341796875, y=w305) -> (x*y=w302:fxp<+/-,34,10>)
    n165 = Select(t=fxp<+,1,1> 0.0, s=w298, f=fxp<+,1,1> 1.0) -> (s? t:f=w300:fxp<+,1,1>)
    n166 = Add(x=w302, y=w295) -> (x+y=w301:fxp<+/-,36,16>)
    n167 = Multiply(x=w301, y=w300) -> (x*y=w296:fxp<+/-,34,18>)
    "fpt_i" <- w296
    n168 = call "Wait"("Count(uSec)"=u32 1000) -> ()  [unwired: 1 out]
  }
  n169 = while "Command type" {
    stop <- FALSE stop-if-true
    n170 = case shown="0, Default" "Command_p" {
      tunnel: ["Dpr_step" w333] -> w330
      frame 0, Default {
        # "Step"
      }
      frame 1 {
        # "Sine"
        n171 = local read "Dpr_sin"() -> (w333:fxp<+/-,22,7>)
      }
    }
    "Dpr_for" <- w330
  }
  n172 = while "All switch" {
    stop <- FALSE stop-if-true
    n173 = case shown="True" "Encoder reset" {
      frame False {
        n174 = local write "Encoder reset_p"(FALSE ("Encoder reset_p")) -> ()
      }
      frame True {
        n175 = flat-sequence {
          frame #0 {
            n176 = local write "Encoder reset_p"(TRUE ("Encoder reset_p")) -> ()
          }
          frame #1 {
            n177 = local write "Encoder reset_p"(FALSE ("Encoder reset_p")) -> ()
          }
        }
      }
    }
  }
  n178 = for {
    N: w8 -> [_]
    tunnel: ["Dp_d_M_avg_Tc (uSec)"] -> w5
    tunnel: [w340] -> w7 mode=indexing
    tunnel: [w339] -> w6 mode=indexing
    n179 = local read "Encoder Position_p1"() -> (w339:i32)
    n180 = call "Wait2"("Count(uSec)"="Dp_d_M_avg_Tc (uSec)") -> ("Tick Count(uSec)"=w340:u32)
  }
  n181 = while "Ini" {
    stop <- FALSE stop-if-true
    n182 = case shown="True" "Ini coe." {
      frame False {
      }
      frame True {
        w346 = i16 2 items=["Backward", "Forward", "Imp"] ("Drive mode")
        w350 = T2 20 items=["50.000 kS/s (NI 9237)"=1, "25.000 kS/s (NI 9237)"=2, "16.667 kS/s (NI 9237)"=3, "12.500 kS/s (NI 9237)"=4, "10.000 kS/s (NI 9237)"=5, "8.333 kS/s (NI 9237)"=6, "7.143 kS/s (NI 9237)"=7, "6.250 kS/s (NI 9237)"=8, "5.556 kS/s (NI 9237)"=9, "5.000 kS/s (NI 9237)"=10, "4.545 kS/s (NI 9237)"=11, "4.167 kS/s (NI 9237)"=12, "3.846 kS/s (NI 9237)"=13, "3.571 kS/s (NI 9237)"=14, "3.333 kS/s (NI 9237)"=15, "3.125 kS/s (NI 9237)"=16, "2.941 kS/s (NI 9237)"=17, "2.778 kS/s (NI 9237)"=18, "2.632 kS/s (NI 9237)"=19, "2.500 kS/s (NI 9237)"=20, "2.381 kS/s (NI 9237)"=21, "2.273 kS/s (NI 9237)"=22, "2.174 kS/s (NI 9237)"=23, "2.083 kS/s (NI 9237)"=24, "2.000 kS/s (NI 9237)"=25, "1.923 kS/s (NI 9237)"=26, "1.852 kS/s (NI 9237)"=27, "1.786 kS/s (NI 9237)"=28, "1.724 kS/s (NI 9237)"=29, "1.667 kS/s (NI 9237)"=30, "1.613 kS/s (NI 9237)"=31] ("Data Rate")
        w365 = i16 0 items=["Step", "Sine"] ("Command_p")
        w366 = i16 2 items=["Raw", "Avg.", "Avg. w. filter"] ("Strain selection_p")
        w367 = fxp<+/-,25,-10> 5.851034075021744e-07  # S/F coeff_p
        n183 = local write "Mag. factor_p"(fxp<+/-,20,3> 1.0 ("Mag. factor_p")) -> ()
        n184 = local write "force_lim"(fxp<+,32,10> 50.0 ("force_lim")) -> ()
        n185 = local write "Kv_p"(fxp<+/-,26,7> 1.0 ("Kv_p")) -> ()
        n186 = local write "S/F coeff_p"(w367) -> ()
        n187 = local write "Data Rate"(w350) -> ()
        n188 = local write "dFp_add"(FALSE ("dFp_add")) -> ()
        n189 = local write "Sin wave freq._p (Hz)"(fxp<+/-,32,6> 1.0 ("Sin wave freq._p (Hz)")) -> ()
        n190 = local write "Sin magnitude_p"(fxp<+/-,21,6> 5.0 ("Sin magnitude_p")) -> ()
        n191 = local write "fp_tolorance"(fxp<+,22,6> 5.0 ("fp_tolorance")) -> ()
        n192 = local write "Sin offset_p"(fxp<+/-,22,7> 0.0 ("Sin offset_p")) -> ()
        n193 = local write "Dpr_step"(fxp<+/-,22,7> 0.0 ("Dpr_step")) -> ()
        n194 = local write "Kp_p"(fxp<+/-,36,9> 30.0 ("Kp_p")) -> ()
        n195 = local write "Kd_p"(fxp<+/-,36,9> 0.0 ("Kd_p")) -> ()
        n196 = local write "Kv_p"(fxp<+/-,22,8> 0.0 ("Kv_p")) -> ()
        n197 = local write "Bv_p"(fxp<+/-,22,8> 0.0 ("Bv_p")) -> ()
        n198 = local write "Ki_p"(fxp<+/-,36,9> 0.0 ("Ki_p")) -> ()
        n199 = local write "Strain selection_p"(w366) -> ()
        n200 = local write "Command_p"(w365) -> ()
        n201 = local write "Drive mode"(w346) -> ()
        n202 = local write "Dp_d_M_avg_Tc (uSec)"(u32 1000 ("D_d_M_avg_Tc (uSec)")) -> ()
        n203 = local write "Belt_out_p"(fxp<+/-,7,7> 36.0 ("Belt_op")) -> ()
        n204 = local write "Belt_in_p"(fxp<+/-,6,6> 16.0 ("Belt_mp")) -> ()
        n205 = local write "mt0_p1"(u32 628319 ("mt0_p1")) -> ()
        n206 = local write "mt0_p2"(u32 628319 ("mt0_p2")) -> ()
      }
    }
  }
  n207 = while "FIFO" {
    stop <- FALSE stop-if-true
    n208 = flat-sequence {
      frame #0 {
        n209 = call "Loop Timer"("Count(uSec)"=u32 1000) -> ()  [unwired: 1 out]
      }
      frame #1 {
        n210 = local read "D_p(mm)"() -> (w377:fxp<+/-,32,7>)
        n211 = local read "Raw Strain_p"() -> (w376:fxp<+/-,36,4>)
        n212 = local read "Strain_p (Avg8)"() -> (w375:fxp<+/-,36,4>)
        n213 = local read "Strain_p (Avg8 w. f)"() -> (w374:fxp<+/-,36,8>)
        n214 = local read "Force_p"() -> (w373:fxp<+/-,32,10>)
        n215 = local read "rad_p1"() -> (w372:fxp<+/-,33,20>)
        n216 = local read "omega_p (T)"() -> (w371:fxp<+/-,36,13>)
        n217 = local read "omega_p (Mavg)"() -> (w370:fxp<+/-,36,13>)
        n218 = Build Array(w377, w376, w375, w374, w373, w372, w371, w370) -> (w378:fxp<+/-,52,20>[])
        n219 = xnode ("FIFO Write")("Element"=w378, "Timeout"=0) -> ()  [unwired: 1 in, 2 out]
      }
    }
  }
  n220 = xnode "FPGA I/O Property Node"("error in"=errorcluster {"status"=FALSE, "code"=0, "source"=""}, "Data Rate"="Data Rate", "Excitation Voltage"="Excitation Voltage") -> ("error out"=w18:errorcluster)  [unwired: 1 in, 1 out]
  n221 = xnode "FPGA I/O Property Node"("error in"=w18, "Half-Bridge Enable"=w13) -> ("error out"=w11:errorcluster)  [unwired: 1 in, 1 out]
  n222 = xnode "FPGA I/O Property Node"("Half-Bridge Enable"=w13) -> ("error out"=w10:errorcluster)  [unwired: 2 in, 1 out]
  n223 = while "Omega_p2 (Mavg)" {
    shift-right: [w381] -> _
    shift-left: w4 -> [w402]
    shift-right: [w382] -> _
    shift-left: w3 -> [w400]
    shift-right: [w386] -> _
    shift-left: _ -> [w384]
    tunnel: w2 -> [w398]
    tunnel: w1 -> [w403]
    stop <- FALSE stop-if-true
    w387 = fxp<+/-,27,3> 3.1415926814079285  # pi
    w390 = fxp<+,32,0> 0.1953125  # 800/4096
    w395 = fxp<+/-,32,0> 0.3183098859153688  # L/2/pi
    n224 = call "Tick Count9"() -> ("Tick Count(uSec)"=w397:u32)
    n225 = Index Array(array=w400, index=0) -> (element=w399:i32)
    n226 = Index Array(array=w402, index=0) -> (element=w401:i32)
    n227 = Multiply(x=w398, y=w403) -> (x*y=w406:i32)
    n228 = Add(x=w406, y=w399) -> (x+y=w405:i32)
    n229 = Greater Or Equal?(x=w397, y=w405) -> (x >= y?=w404:bool)
    n230 = case shown="True" w404 {
      tunnel: w402 -> [w410 w425]
      tunnel: w401 -> [_ w417]
      tunnel: w400 -> [w411 w426]
      tunnel: w399 -> [_ w427]
      tunnel: w398 -> [_ w424]
      tunnel: w397 -> [_ w412]
      tunnel: [w410 w415] -> w381
      tunnel: [w411 w414] -> w382
      tunnel: [w409 w413] -> w386
      tunnel: w384 -> [w409 _]
      frame False {
      }
      frame True {
        n231 = local read "Encoder Position_p2"() -> (w416:i32)
        n232 = Subtract(x=w412, y=w427) -> (x-y=w428:u32)
        n233 = Insert Into Array(array=w426, new element=w412) -> (w430:i32[])  [unwired: 1 in]
        n234 = Subtract(x=w416, y=w417) -> (x-y=w421:i32)
        n235 = Insert Into Array(array=w425, index=w424, new element=w416) -> (w431:i32[])
        n236 = To Fixed-Point(number=w428) -> (fixed-point=w418:fxp<+,32,32>)  [unwired: 1 in]
        n237 = Multiply(x=w421, y=2500) -> (x*y=w422:i32)
        n238 = To Fixed-Point(number=w422) -> (fixed-point=w423:fxp<+/-,32,32>)  [unwired: 1 in]
        n239 = Delete From Array(array=w430, length=1, index=0) -> (array with subset deleted=w414:i32[])  [unwired: 1 out]
        n240 = Delete From Array(array=w431, length=1, index=0) -> (array with subset deleted=w415:i32[])  [unwired: 1 out]
        n241 = Divide(x=w423, y=w418) -> (x/y=w413:fxp<+/-,64,32>)
      }
    }
    n242 = local read "Mag. factor_p"() -> (w389:fxp<+/-,20,3>)
    n243 = local read "Belt_in_p"() -> (w392:fxp<+/-,6,6>)
    n244 = local read "Belt_out_p"() -> (w391:fxp<+/-,7,7>)
    n245 = Divide(x=w390, y=w389) -> (x/y=w380:fxp<+/-,32,1>)
    n246 = Multiply(x=w387, y=w386) -> (x*y=w388:fxp<+/-,64,35>)
    n247 = Multiply(x=w395, y=w392) -> (x*y=w396:fxp<+/-,38,6>)
    n248 = Multiply(x=w380, y=w388) -> (x*y=w383:fxp<+/-,64,36>)
    "omega_p2 (Mavg)" <- w383
    n249 = Divide(x=w396, y=w391) -> (x/y=w394:fxp<+/-,45,6>)
    n250 = Multiply(x=w394, y=w383) -> (x*y=→"Dp2_d (Mavg)":fxp<+/-,64,41>)
  }
  n251 = while "Omega_p1 (Mavg)" {
    tunnel: w8 -> [w452]
    shift-right: [w450] -> _
    shift-left: w7 -> [w455]
    shift-right: [w449] -> _
    shift-left: w6 -> [w451]
    shift-right: [w448] -> _
    shift-left: _ -> [w447]
    tunnel: w5 -> [w445]
    stop <- FALSE stop-if-true
    w439 = fxp<+/-,27,3> 3.1415926814079285  # pi
    w438 = fxp<+/-,32,0> 0.3183098859153688  # L/2/pi
    n252 = call "Tick Count5"() -> ("Tick Count(uSec)"=w456:u32)
    n253 = Index Array(array=w455, index=0) -> (element=w454:u32)
    n254 = Index Array(array=w451, index=0) -> (element=w453:i32)
    n255 = Multiply(x=w452, y=w445) -> (x*y=w458:i32)
    n256 = Add(x=w458, y=w454) -> (x+y=w457:u32)
    n257 = Greater Or Equal?(x=w456, y=w457) -> (x >= y?=w446:bool)
    n258 = case shown="True" w446 {
      tunnel: w456 -> [_ w479]
      tunnel: w452 -> [_ w476]
      tunnel: w455 -> [w463 w478]
      tunnel: w454 -> [_ w477]
      tunnel: w453 -> [_ w473]
      tunnel: w451 -> [w462 w475]
      tunnel: [w461 w471] -> w448
      tunnel: [w463 w470] -> w450
      tunnel: [w462 w469] -> w449
      tunnel: w447 -> [w461 _]
      frame False {
      }
      frame True {
        n259 = local read "Encoder Position_p1"() -> (w472:i32)
        n260 = Subtract(x=w479, y=w477) -> (x-y=w480:u32)
        n261 = Subtract(x=w472, y=w473) -> (x-y=w465:i32)
        n262 = Insert Into Array(array=w478, new element=w479) -> (w482:u32[])  [unwired: 1 in]
        n263 = Insert Into Array(array=w475, index=w476, new element=w472) -> (w483:i32[])
        n264 = To Fixed-Point(number=w480) -> (fixed-point=w467:fxp<+,32,32>)  [unwired: 1 in]
        n265 = Multiply(x=w465, y=2500) -> (x*y=w466:i32)
        n266 = To Fixed-Point(number=w466) -> (fixed-point=w474:fxp<+/-,32,32>)  [unwired: 1 in]
        n267 = Delete From Array(array=w482, length=1, index=0) -> (array with subset deleted=w470:u32[])  [unwired: 1 out]
        n268 = Delete From Array(array=w483, length=1, index=0) -> (array with subset deleted=w469:i32[])  [unwired: 1 out]
        n269 = Divide(x=w474, y=w467) -> (x/y=w471:fxp<+/-,64,32>)
      }
    }
    n270 = local read "Belt_in_p"() -> (w443:fxp<+/-,6,6>)
    n271 = local read "Belt_out_p"() -> (w442:fxp<+/-,7,7>)
    n272 = Multiply(x=w439, y=w448) -> (x*y=w444:fxp<+/-,64,35>)
    n273 = Multiply(x=w438, y=w443) -> (x*y=w441:fxp<+/-,38,6>)
    n274 = Multiply(x=fxp<+/-,2,2> 1.0 ("f"), y=w444) -> (x*y=w437:fxp<+/-,64,37>)
    "omega_p1 (Mavg)" <- w437
    n275 = Divide(x=w441, y=w442) -> (x/y=w436:fxp<+/-,45,6>)
    n276 = Multiply(x=w436, y=w437) -> (x*y=→"Dp1_d (Mavg)":fxp<+/-,64,42>)
  }
  n277 = Merge Errors(w11, w10) -> (w12:errorcluster)
  n278 = xnode "FPGA I/O Node"("error in"=w12, "Mod6/Start"=TRUE) -> ("error out"=w16:errorcluster)  [unwired: 1 in, 1 out]
  n279 = while "PID force controller_p" {
    shift-right: [w490] -> _
    shift-left: _ -> [w489]
    stop <- FALSE stop-if-true
    n280 = local read "Force_p"() -> (w502:fxp<+/-,32,10>)
    n281 = local read "fpt_d"() -> (w498:fxp<+/-,36,18>)
    n282 = local read "Fr_p"() -> (w503:fxp<+/-,32,10>)
    n283 = Subtract(x=w503, y=w502) -> (x-y=w500:fxp<+/-,33,11>)
    "fp_tilde" <- w500
    n284 = local read "fpt_i"() -> (w494:fxp<+/-,34,18>)
    n285 = Multiply(x="Kp_p", y=w500) -> (x*y=w496:fxp<+/-,64,23>)
    n286 = Multiply(x="Kd_p", y=w498) -> (x*y=w497:fxp<+/-,64,27>)
    n287 = Absolute Value(x=w500) -> (abs(x)=w509:fxp<+,32,10>)
    n288 = Add(x=w496, y=w497) -> (x+y=w492:fxp<+/-,64,28>)
    n289 = Multiply(x="Ki_p", y=w494) -> (x*y=w493:fxp<+/-,64,27>)
    n290 = call "Tick Count7"() -> ("Tick Count(uSec)"=w490:u32)
    n291 = Add(x=w492, y=w493) -> (x+y=w491:fxp<+/-,64,29>)
    n292 = Greater?(x=w509, y="fp_tolorance") -> (0:w506:bool)
    n293 = Subtract(x=w490, y=w489) -> (x-y=w488:u32)
    n294 = Divide(x=u32 1000, y=w488) -> (x/y=→"PID (kHz)":fxp<+/-,20,7>)
    n295 = Select(t=w491, s=w506, f=fxp<+,1,1> 0.0) -> (s? t:f=→"Fp_PID":fxp<+/-,64,29>)
  }
  n296 = while "Protection" {
    stop <- FALSE stop-if-true
    n297 = local read "Force_p"() -> (w514:fxp<+/-,32,10>)
    n298 = Absolute Value(x=w514) -> (abs(x)=w513:fxp<+,32,10>)
    n299 = Greater?(x=w513, y="force_lim") -> (0:w511:bool)
    n300 = case shown="True" w511 {
      frame False {
      }
      frame True {
        n301 = local write "Stop motor_p"(TRUE ("Stop motor_p")) -> ()
      }
    }
  }
  n302 = while "ft_d" {
    stop <- FALSE stop-if-true
    n303 = local read "Dp_error_dd"() -> (w522:fxp<+/-,36,16>)
    n304 = local read "Dp_error_d"() -> (w524:fxp<+/-,33,8>)
    n305 = local read "Kv_p"() -> (w525:fxp<+/-,26,7>)
    n306 = local read "Bv_p"() -> (w523:fxp<+/-,22,8>)
    n307 = Multiply(x=w524, y=w525) -> (x*y=w520:fxp<+/-,59,15>)
    n308 = Multiply(x=w522, y=w523) -> (x*y=w521:fxp<+/-,58,24>)
    n309 = local read "Force_p"() -> (w518:fxp<+/-,32,10>)
    n310 = Add(x=w520, y=w521) -> (x+y=w519:fxp<+/-,64,24>)
    n311 = Subtract(x=w519, y=w518) -> (x-y=→"fpt_d":fxp<+/-,64,25>)
  }
  n312 = while "Derivative" {
    stop <- FALSE stop-if-true
    n313 = local read "Dpr_sin_dd"() -> (w534:fxp<+/-,35,20>)
    n314 = local read "Dpr_sin_d"() -> (w536:fxp<+/-,33,15>)
    n315 = local read "Stop motor_p"() -> (w532:bool)
    n316 = local read "Dp_error"() -> (w537:fxp<+/-,22,7>)
    n317 = local read "Dp_dd"() -> (w535:fxp<+/-,36,25>)
    n318 = Subtract(x=w536, y=w537) -> (x-y=w529:fxp<+/-,34,16>)
    n319 = Subtract(x=w534, y=w535) -> (x-y=w533:fxp<+/-,41,26>)
    n320 = Select(t=fxp<+,1,1> 0.0, s=w532, f=w529) -> (s? t:f=→"Dp_error_d":fxp<+/-,34,16>)
    n321 = Select(t=fxp<+/-,41,26> 0.0, s=w532, f=w533) -> (s? t:f=→"Dp_error_dd":fxp<+/-,41,26>)
  }
  n322 = while "Omega_p(T method)" {
    shift-right: [w569] -> _
    shift-left: _ -> [w567]
    shift-right: [w550] -> _
    shift-left: _ -> [w568]
    shift-right: [w565] -> _
    shift-left: _ -> [w566]
    shift-right: [w543] -> _
    shift-left: _ -> [w542]
    shift-right: [w538] -> _
    shift-left: _ -> [w540]
    shift-right: [w546] -> _
    shift-left: _ -> [w545]
    stop <- FALSE stop-if-true
    w557 = fxp<+/-,32,0> 0.3183098859153688  # L/2/pi
    w562 = fxp<+/-,32,0> 0.3183098859153688  # L/2/pi
    n323 = local read "Encoder Position_p1"() -> (w569:i32)
    n324 = local read "Encoder Position_p2"() -> (w543:i32)
    n325 = call "Tick Count4"() -> ("Tick Count(Ticks)"=w544:u32)
    n326 = call "omega_sub_Encoder_800ppr.vi"("mt0"="mt0_p1", "omega_pre"=w568, "ticks_m_pre"=w566, "ticks"=w544, "count_pre"=w567, "count"=w569) -> ("ticks_m"=w565:u32, "mt"=→"mt_omega_p1":u32, "omega"=w550:fxp<+/-,36,13>)  [unwired: 3 in]
    "omega_p1 (T)" <- w550
    n327 = call "omega_sub_Encoder_4096ppr.vi"("mt0"="mt0_p2", "omega_pre"=w540, "ticks_m_pre"=w545, "ticks"=w544, "count_pre"=w542, "count"=w543) -> ("ticks_m"=w546:u32, "mt"=→"mt_omega_p2":u32, "omega"=w538:fxp<+/-,36,13>)  [unwired: 3 in]
    n328 = local read "Mag. factor_p"() -> (w558:fxp<+/-,20,3>)
    n329 = local read "Belt_in_p"() -> (w555:fxp<+/-,6,6>)
    n330 = local read "Belt_out_p"() -> (w554:fxp<+/-,7,7>)
    n331 = Multiply(x=w562, y="Belt_in_p") -> (x*y=w560:fxp<+/-,38,6>)
    n332 = Multiply(x=w557, y=w555) -> (x*y=w556:fxp<+/-,38,6>)
    n333 = Divide(x=w560, y="Belt_out_p") -> (x/y=w551:fxp<+/-,20,1>)
    n334 = Divide(x=w538, y=w558) -> (x/y=w539:fxp<+/-,57,31>)
    "omega_p2 (T)" <- w539
    n335 = Divide(x=w556, y=w554) -> (x/y=w549:fxp<+/-,45,6>)
    n336 = Multiply(x=w549, y=w539) -> (x*y=→"Dp2_d (T)":fxp<+/-,36,13>)
    n337 = Multiply(x=w551, y=w550) -> (x*y=→"Dp1_d (T)":fxp<+/-,36,13>)
  }
  n338 = while {
    tunnel: [w570] -> w9
    shift-right: [w594] -> _
    shift-left: _ -> [w595]
    tunnel: w16 -> [w590]
    shift-right: [w586] -> _
    shift-left: _ -> [w587]
    shift-right: [w582] -> _
    shift-left: _ -> [w581]
    shift-right: [w581] -> _
    shift-left: _ -> [w580]
    shift-right: [w580] -> _
    shift-left: _ -> [w579]
    shift-right: [w579] -> _
    shift-left: _ -> [w578]
    shift-right: [w578] -> _
    shift-left: _ -> [w577]
    shift-right: [w577] -> _
    shift-left: _ -> [w576]
    shift-right: [w576] -> _
    shift-left: _ -> [w575]
    stop <- w589 stop-if-true
    w584 = fxp<+,20,2> 2.115001678466797  # Gage Factor
    n339 = xnode "FPGA I/O Node"("error in"=w590) -> ("error out"=w570:errorcluster, "Mod6/AI3"=w585:fxp<+/-,24,-4>)  [unwired: 1 in, 1 out]
    n340 = Select(t=w585, s="Strain gage reset_p", f=w587) -> (s? t:f=w586:fxp<+/-,24,-4>)
    n341 = Or(x="Stop (Strain)", y=w570) -> (x .or. y?=w589:bool)
    n342 = Subtract(x=w585, y=w586) -> (x-y=w583:fxp<+/-,30,-3>)
    "Mod6/AI3" <- w583
    n343 = Multiply(x=w584, y=w583) -> (x*y=w582:fxp<+/-,50,-1>)
    "Raw Strain_p" <- w582
    n344 = call "average_v2.vi"("Numeric 8"=w575, "Numeric"=w582, "Numeric 7"=w576, "Numeric 2"=w581, "Numeric 6"=w577, "Numeric 5"=w578, "Numeric 4"=w579, "Numeric 3"=w580) -> ("Mean (8pt)"=w574:fxp<+/-,32,4>)  [unwired: 1 in, 2 out]
    "Strain_p (Avg8)" <- w574
    n345 = call "Tick Count"() -> ("Tick Count(uSec)"=w594:u32)
    n346 = xnode "Butterworth Filter"("input data"=w574, "scaled coefficients"="Strain_p Avg.8 coeff.") -> ("output data"=→"Strain_p (Avg8 w. f)":fxp<+/-,36,8>)  [unwired: 1 in]
    n347 = Subtract(x=w594, y=w595) -> (x-y=w593:fxp<+/-,32,16>)
    n348 = Divide(x=fxp<+,7,10> 1000.0, y=w593) -> (x/y=→"Loop rate (kHz)":fxp<+/-,40,27>)
  }
  n349 = while "Mechanism parameter (Ptich)" {
    stop <- FALSE stop-if-true
    n350 = local read "D_p(mm)"() -> (w655:fxp<+/-,32,7>)
    n351 = local read "r4p"() -> (w652:fxp<+/-,32,9>)
    n352 = local read "r4p"() -> (w648:fxp<+/-,32,9>)
    n353 = local read "r4p"() -> (w629:fxp<+/-,32,9>)
    n354 = local read "r4p"() -> (w632:fxp<+/-,32,9>)
    n355 = local read "r4p"() -> (w649:fxp<+/-,32,9>)
    n356 = Square(x=w652) -> (x^2=w651:fxp<+,63,17>)
    n357 = local read "r4p"() -> (w633:fxp<+/-,32,9>)
    n358 = Square(x=w648) -> (x^2=w647:fxp<+,63,17>)
    n359 = Add(x=fxp<+,26,7> 84.26000022888184, y=w655) -> (x+y=→"r4p":fxp<+/-,34,9>)
    n360 = Square(x=w632) -> (x^2=w631:fxp<+,63,17>)
    n361 = Square(x=w629) -> (x^2=w628:fxp<+,63,17>)
    n362 = Multiply(x=fxp<+,6,6> 49.0, y=w649) -> (x*y=w643:fxp<+/-,38,15>)
    n363 = Add(x=fxp<+/-,29,14> -5537.627593994141, y=w651) -> (x+y=w641:fxp<+/-,63,17>)
    n364 = Add(x=fxp<+/-,29,14> -7099.747589111328, y=w647) -> (x+y=w645:fxp<+/-,63,17>)
    n365 = Multiply(x=fxp<+,36,8> 161.07878321036696, y=w633) -> (x*y=w614:fxp<+/-,64,17>)
    n366 = Subtract(x=fxp<+/-,32,14> -4126.81995010376, y=w631) -> (x-y=w624:fxp<+/-,64,18>)
    n367 = Subtract(x=fxp<+/-,30,15> -9526.889709472656, y=w628) -> (x-y=w626:fxp<+/-,64,18>)
    n368 = Square(x=w643) -> (x^2=w609:fxp<+,64,28>)
    n369 = Multiply(x=w641, y=w645) -> (x*y=w608:fxp<+/-,64,33>)
    n370 = Multiply(x=w624, y=w626) -> (x*y=w605:fxp<+,64,33>)
    n371 = Multiply(x=w614, y=w614) -> (x*y=w606:fxp<+/-,64,34>)
    n372 = Subtract(x=w609, y=w608) -> (x-y=w611:fxp<+,64,35>)
    n373 = Subtract(x=w609, y=w608) -> (x-y=→"(b^2-ac)p2":fxp<+/-,64,34>)
    n374 = Subtract(x=w606, y=w605) -> (x-y=w616:fxp<+,64,20>)
    n375 = xnode "High Throughput Square Root"("x"=w611) -> ("sqrt(x)"=w610:fxp<+,33,18>)
    n376 = Negate(x=w643) -> (-x=w644:fxp<+/-,38,15>)
    n377 = Subtract(x=fxp<+/-,64,40> 0.0, y=w614) -> (x-y=w612:fxp<+/-,64,17>)
    n378 = Subtract(x=w606, y=w605) -> (x-y=→"(b^2-ac)p3":fxp<+/-,64,35>)
    n379 = xnode "High Throughput Square Root"("x"=w616) -> ("sqrt(x)"=w615:fxp<+,32,10>)
    n380 = Add(x=w644, y=w610) -> (x+y=w642:fxp<+/-,43,20>)
    n381 = Add(x=w612, y=w615) -> (x+y=w625:fxp<+/-,64,18>)
    n382 = Divide(x=w642, y=w641) -> (x/y=w640:fxp<+/-,64,66>)
    n383 = Divide(x=w625, y=w624) -> (x/y=w623:fxp<+/-,64,7>)
    n384 = To Fixed-Point(number=w640) -> (fixed-point=w639:fxp<+/-,64,66>)  [unwired: 1 in]
    n385 = To Fixed-Point(number=w623) -> (fixed-point=w622:fxp<+/-,64,7>)  [unwired: 1 in]
    n386 = xnode "High Throughput Inverse Tangent (2 Input)"("y"=w639, "x"=fxp<+/-,32,16> 1.0) -> ("atan2(y,x) (pi)"=w636:fxp<+/-,16,2>)
    n387 = xnode "High Throughput Inverse Tangent (2 Input)"("y"=w622, "x"=fxp<+/-,32,16> 1.0) -> ("atan2(y,x) (pi)"=w620:fxp<+/-,16,2>)
    n388 = Multiply(x=w636, y=fxp<+,1,2> 2.0) -> (x*y=→"theta2p (rad)":fxp<+/-,16,3>)
    n389 = Multiply(x=w620, y=fxp<+/-,3,3> 2.0) -> (x*y=→"theta3p (rad)":fxp<+/-,19,5>)
  }
  n390 = while {
    stop <- FALSE stop-if-true
    n391 = local read "omega_p1 (Mavg)"() -> (w764:fxp<+/-,36,14>)
    n392 = local read "Dp1_d (Mavg)"() -> (w760:fxp<+/-,36,14>)
    n393 = call "Loop Timer2"("Count(uSec)"="Mavg f loop(uSec)") -> ()  [unwired: 1 out]
    n394 = xnode "Butterworth Filter"("input data"=w764, "scaled coefficients"="omega_P(Mavg) coeff.") -> ("output data"=→"omega_p (Mavg w. f)":fxp<+/-,36,18>)  [unwired: 1 in]
    n395 = xnode "Butterworth Filter"("input data"=w760, "scaled coefficients"="Dp_d (Mavg) coeff.") -> ("output data"=→"Dp_d (Mavg w. f.)":fxp<+/-,36,18>)  [unwired: 1 in]
  }
  n396 = while "Quadrature drive_p" {
    stop <- FALSE stop-if-true
    n397 = local read "Drive mode"() -> (w782:i16)
    n398 = case shown="2" w782 {
      tunnel: [w792 w793 w794] -> w781
      frame 0, Default {
        # "Backward"
        n399 = local read "Fp_PID"() -> (w792:fxp<+/-,36,16>)
      }
      frame 1 {
        # "Forward"
        n400 = local read "Fr_p"() -> (w793:fxp<+/-,32,10>)
      }
      frame 2 {
        # "Imp"
        n401 = local read "Fp_PID"() -> (w794:fxp<+/-,36,16>)
      }
    }
    n402 = local read "dFp_PID"() -> (w785:fxp<+/-,36,18>)
    n403 = local read "omega_p (rad/s)"() -> (w789:fxp<+/-,36,13>)
    n404 = Select(t=w785, s="dFp_add", f=fxp<+,1,1> 0.0) -> (s? t:f=w788:fxp<+/-,36,18>)
    n405 = call "Oriental_step_motor_PKP225.vi"("F_Threshold"="F_Threshold_p", "dFmr"=w788, "omega"=w789, "Fmr"=w781) -> ("vq_F"=→"vq_p_F":fxp<+/-,36,9>, "vd_F"=→"vd_p_F":fxp<+/-,36,9>)  [unwired: 6 in]
  }
  n406 = while "Force to torque" {
    stop <- FALSE stop-if-true
    w802 = fxp<+,16,-5> 0.024499893188476562  # r2p
    n407 = local read "theta3p (rad)"() -> (w805:fxp<+/-,19,5>)
    n408 = local read "theta2p (rad)"() -> (w804:fxp<+/-,16,2>)
    n409 = Subtract(x=w805, y=w804) -> (x-y=w803:fxp<+/-,19,5>)
    n410 = xnode "High Throughput Sine & Cosine"("x (pi)"=w803) -> ("sin(x)"=w801:fxp<+/-,16,2>)  [unwired: 1 out]
    n411 = local read "Force_p"() -> (w800:fxp<+/-,32,10>)
    n412 = Multiply(x=w802, y=w801) -> (x*y=w797:fxp<+/-,32,-3>)
    n413 = Divide(x="kv_p (Nm/rad)", y=w797) -> (x/y=w795:fxp<+/-,64,43>)
    n414 = Multiply(x=w797, y=w800) -> (x*y=→"tau_p (Nm)":fxp<+/-,63,6>)
    n415 = local write "Kv_p"(w795) -> ()
  }
  n416 = xnode "FPGA I/O Node"("error in"=w9, "Mod6/Stop"=TRUE) -> ()  [unwired: 1 in, 2 out]
